vi "Eulogy Date.vi"(8 "Error In":errorcluster, 10 "Tag Length":i32=5, 11 "Label Text":string) -> (0 "Error Out":errorcluster, 3 "Date":string)   [LabVIEW 2017, in "Graveyard.lvlib"]
uses:
  Graveyard.lvlib
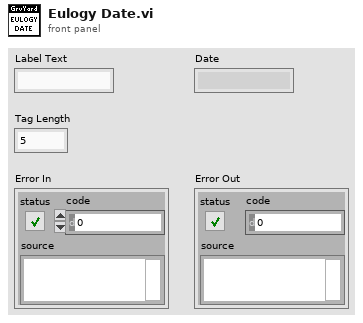
[diagram p1: front panel]
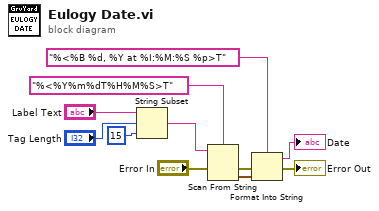
[diagram p0: block diagram]
diagram:
  n1 = String Subset(string="Label Text", offset (0)="Tag Length", length (rest)=15 ("length (rest)")) -> (substring=w4:string)
  n2 = Scan From String(format string="%<%Y%m%dT%H%M%S>T", input string=w4, error in="Error In") -> (error out=w7:errorcluster, output 1=w10:timestamp)  [unwired: 2 in, 2 out]
  n3 = Format Into String(format string="%<%B %d, %Y at %I:%M:%S %p>T", error in=w7, w10) -> (resulting string=→"Date":string, error out=→"Error Out":errorcluster)  [unwired: 1 in]
